vi "Anti-Tilt.vi"(8 "Lateral - X":dbl, 11 "Longitudinal - Y":dbl) -> (0 "Lateral - X":dbl, 3 "Longitudinal - Y":dbl)   [LabVIEW 2018]
panel:
  out "Connected":bool
  out "YRPHfH":T1
  # "Pitch and Roll are swapped inside the VI."
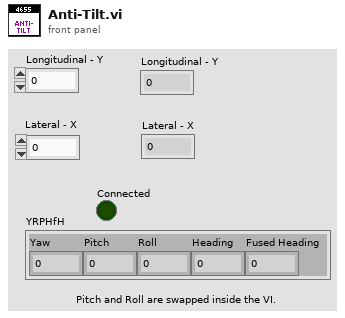
[diagram p1: front panel]
types:
  T1 = cluster{"Yaw":dbl, "Pitch":dbl, "Roll":dbl, "Heading":dbl, "Fused Heading":dbl}
  T2 = cluster{"Yaw":dbl, "Roll":dbl, "Pitch":dbl, "Heading":dbl, "Fused Heading":dbl}
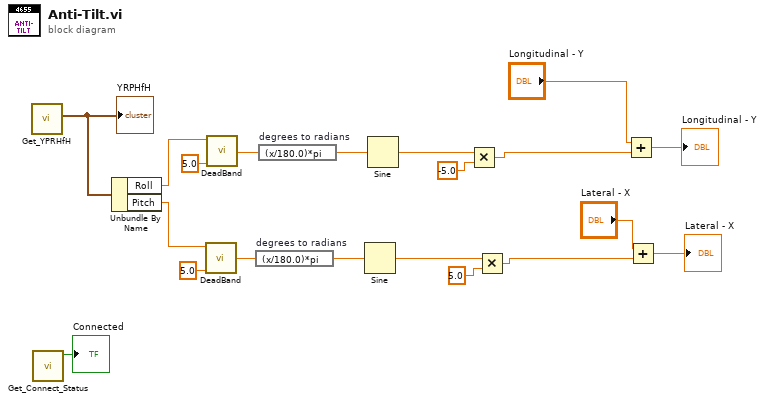
[diagram p0: block diagram]
diagram:
  n1 = call <vilib>:"Get_YPRHfH.vi"() -> ("YRPHfH"=w20:T2)  [unwired: 11 in]
  "YRPHfH" <- w20
  n2 = call <vilib>:"Get_Connect_Status.vi"() -> ("Connected"=→"Connected":bool)  [unwired: 11 in]
  n3 = Unbundle By Name(w20) -> ("Roll"=w14:dbl, "Pitch"=w15:dbl)
  n4 = call "DeadBand.vi"("Deadband"=5.0, "Input"=w15) -> ("Output"=w11:dbl)  [unwired: 9 in]
  n5 = call "DeadBand.vi"("Deadband"=5.0, "Input"=w14) -> ("Output"=w13:dbl)  [unwired: 9 in]
  n6 = expression code="(x/180.0)*pi" "degrees to radians"(w11) -> (w10:dbl)
  n7 = expression code="(x/180.0)*pi" "degrees to radians"(w13) -> (w12:dbl)
  n8 = Sine(x=w10) -> (sin(x)=w8:dbl)
  n9 = Sine(x=w12) -> (sin(x)=w19:dbl)
  n10 = Multiply(x=w19, y=-5.0) -> (x*y=w9:dbl)
  n11 = Multiply(x=w8, y=5.0) -> (x*y=w7:dbl)
  n12 = Add(x="Longitudinal - Y", y=w9) -> (x+y=→"Longitudinal - Y":dbl)
  n13 = Add(x="Lateral - X", y=w7) -> (x+y=→"Lateral - X":dbl)
